vi "Control Example.vi"() -> ()   [LabVIEW 2016]
doc: "Demonstrates the Control Menu type. Right click on the \"Listbox\" to see the menu generated.\n\nClick summarys show up in the history array. Click the \"Add Item\" to add a dummy item to the control's menu."
uses:
  <userlib>/_MGI/Menu Building/SelectionType/RadioSelection/MGI_RadioSelection.lvclass
  C:/Program Files (x86)/National Instruments/LabVIEW 2016/user.lib/_MGI/Menu Building/SelectionType/MGI_SelectionType.lvclass
  <userlib>/_MGI/Menu Building/SelectionType/CheckmarkSelection/MGI_CheckmarkSelection.lvclass
  <userlib>/_MGI/Menu Building/MenuItem/MenuSeparatorItem/MGI_MenuSeparatorItem.lvclass
  C:/Program Files (x86)/National Instruments/LabVIEW 2016/user.lib/_MGI/Menu Building/MenuItem/MGI_MenuItem.lvclass
  <userlib>/_MGI/Menu Building/MenuTypes/Control/MGI_Control.lvclass
  C:/Program Files (x86)/National Instruments/LabVIEW 2016/user.lib/_MGI/Menu Building/MenuTypes/MGI_Menu.lvclass
  <userlib>/_MGI/Menu Building/MenuItem/MenuItem.vi
  <userlib>/_MGI/Menu Building/SelectionType/RadioSelection/RadioSelection.vi
  <userlib>/_MGI/Menu Building/MenuItem/Write Click By Default.vi
  <userlib>/_MGI/Menu Building/MenuItem/Write Sub-Menus.vi
  <userlib>/_MGI/Menu Building/MenuTypes/Control/Control.vi
  <userlib>/_MGI/Menu Building/SelectionType/CheckmarkSelection/CheckmarkSelection.vi
  <userlib>/_MGI/Menu Building/MenuItem/MenuSeparatorItem/MenuSeparatorItem.vi
  <userlib>/_MGI/Menu Building/MenuTypes/Read Menu Items.vi
  <userlib>/_MGI/Menu Building/MenuItem/MGI_MenuItem.lvclass
  <userlib>/_MGI/Menu Building/SelectionType/MGI_SelectionType.lvclass
  <userlib>/_MGI/Menu Building/MenuTypes/MGI_Menu.lvclass
  <userlib>/_MGI/Menu Building/MenuItemStatusChange/MGI_MenuItemStatusChange.lvclass
panel:
  out "History 2":T1(array[cluster])
  in  "Listbox 2":i32(listbox)
  out "History":T1(array[cluster])
  in  "Add Item":bool
  in  "stop":bool
  in  "Listbox":i32(listbox)
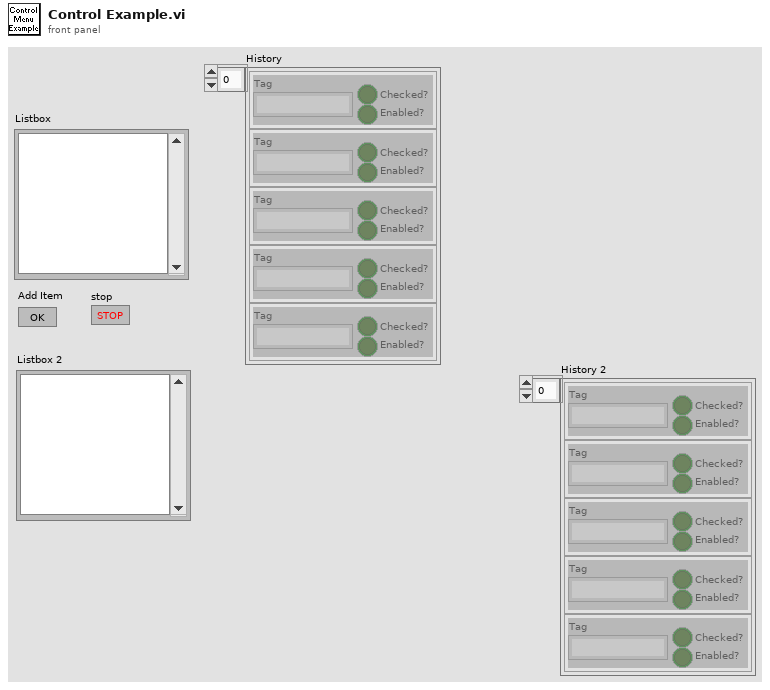
[diagram p1: front panel]
types:
  T1 = cluster{"Tag":string, "Checked?":bool, "Enabled?":bool}[]
  T2 = cluster{"Tag":string, "Checked?":bool, "Enabled?":bool}
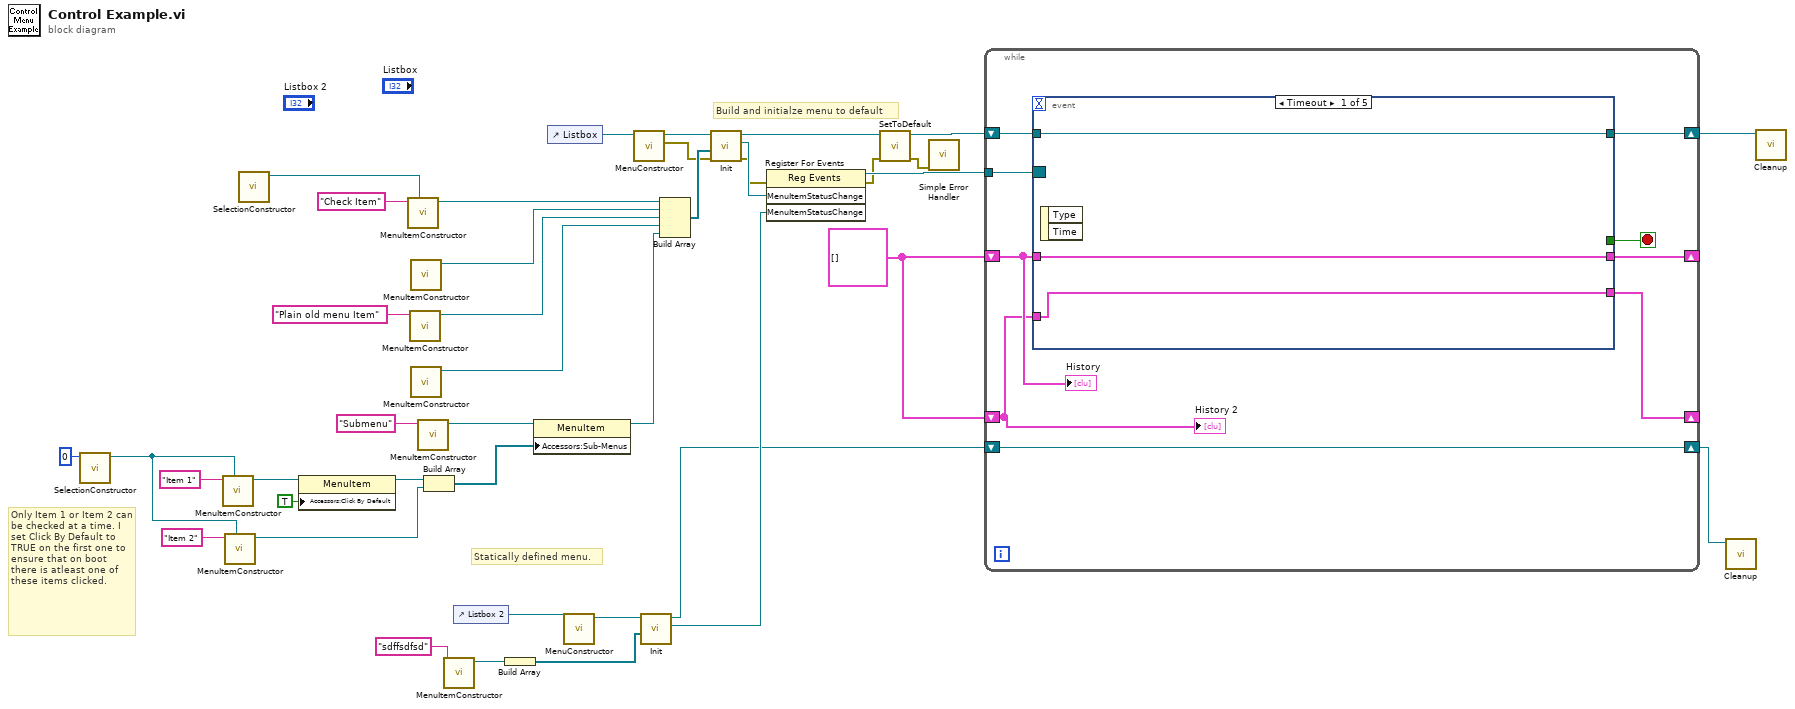
[diagram p0: block diagram]
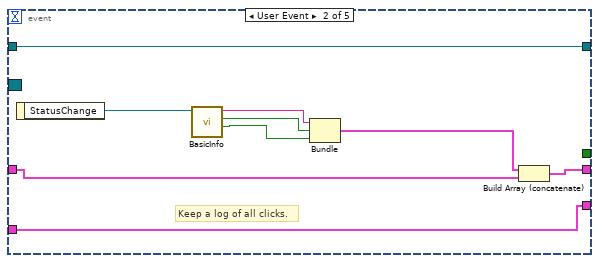
[diagram p2: hidden frame]
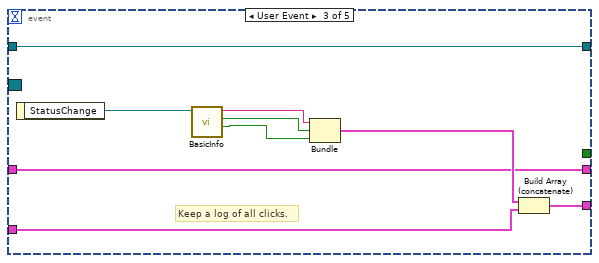
[diagram p3: hidden frame]
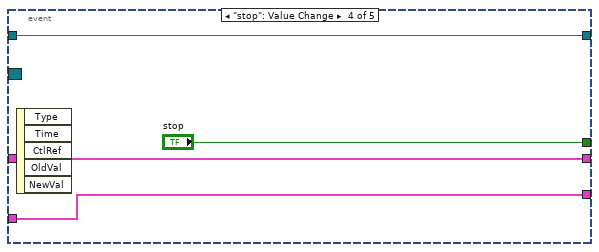
[diagram p4: hidden frame]
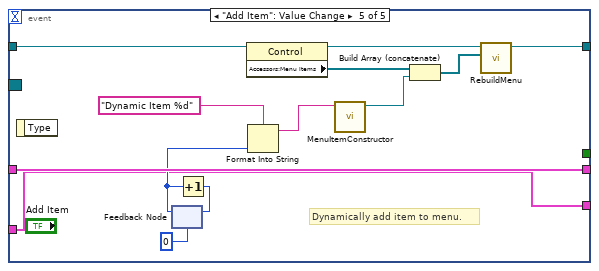
[diagram p5: hidden frame]
diagram:
  w7 = T1 [] ("Array")
  # "Build and initialze menu to default"
  # "Only Item 1 or Item 2 can be checked at a time. I set Click By Default to TRUE on the first one to ensure that on boot there is atleast one of these items clicked."
  # "Statically defined menu."
  n1 = call-poly <userlib>:"SelectionConstructor.vi"("Group"=u8 0) -> ("RadioSelection out"=w26:refnum<class "MGI_RadioSelection.lvclass">)  [unwired: 9 in, 1 out]
  n2 = call-poly <userlib>:"MenuItemConstructor.vi"("Selection Type"=w26, "Text"="Item 1") -> ("MenuItem"=w29:refnum<data-value>)  [unwired: 8 in, 1 out]
  n3 = call-poly <userlib>:"MenuItemConstructor.vi"("Selection Type"=w26, "Text"="Item 2") -> ("MenuItem"=w28:refnum<data-value>)  [unwired: 8 in, 1 out]
  n4 = call-poly <userlib>:"SelectionConstructor.vi"() -> ("CheckmarkSelection out"=w35:refnum<class "MGI_CheckmarkSelection.lvclass">)  [unwired: 10 in, 1 out]
  n5 = property class="MenuItem"(reference=w29, "Accessors:Click By Default"=TRUE ("Click By Default")) -> (reference out=w21:refnum<data-value>)  [unwired: 1 in, 1 out]
  n6 = call-poly <userlib>:"MenuItemConstructor.vi"("Selection Type"=w35, "Text"="Check Item") -> ("MenuItem"=w37:refnum<data-value>)  [unwired: 8 in, 1 out]
  n7 = call-poly <userlib>:"MenuItemConstructor.vi"("Text"="Plain old menu Item") -> ("MenuItem"=w1:refnum<data-value>)  [unwired: 9 in, 1 out]
  n8 = call-poly <userlib>:"MenuItemConstructor.vi"() -> ("MenuSeparatorItem"=w22:refnum<data-value>)  [unwired: 10 in, 1 out]
  n9 = call-poly <userlib>:"MenuItemConstructor.vi"() -> ("MenuSeparatorItem"=w3:refnum<data-value>)  [unwired: 10 in, 1 out]
  n10 = call-poly <userlib>:"MenuItemConstructor.vi"("Text"="Submenu") -> ("MenuItem"=w32:refnum<data-value>)  [unwired: 9 in, 1 out]
  n11 = Build Array(w21, w28) -> (w27:refnum<data-value>[])
  n12 = call-poly <userlib>:"MenuItemConstructor.vi"("Text"="sdffsdfsd") -> ("MenuItem"=w10:refnum<data-value>)  [unwired: 9 in, 1 out]
  n13 = control-ref of="Listbox 2"() -> (w14:refnum<vi>)
  n14 = Build Array(w10) -> (w9:refnum<data-value>[])
  n15 = property class="MenuItem"(reference=w32, "Accessors:Sub-Menus"=w27) -> (reference out=w33:refnum<data-value>)  [unwired: 1 in, 1 out]
  n16 = control-ref of="Listbox"() -> (w24:refnum<vi>)
  n17 = call-poly <userlib>:"MenuConstructor.vi"("Ctl Refnum"=w14) -> ("Control out"=w15:refnum<class "MGI_Control.lvclass">)  [unwired: 9 in, 1 out]
  n18 = call-poly <userlib>:"MenuConstructor.vi"("Ctl Refnum"=w24) -> ("error out"=w6:errorcluster, "Control out"=w23:refnum<class "MGI_Control.lvclass">)  [unwired: 9 in]
  n19 = call-dynamic "Init.vi"("Menu Items"=w9, "Menu in"=w15) -> ("MenuItemStatusChange"=w13:refnum<user-event>, "Menu out"=w12:refnum<class "MGI_Control.lvclass">)  [unwired: 7 in, 1 out]
  n20 = Build Array(w37, w22, w1, w3, w33) -> (w40:refnum<data-value>[])
  n21 = call-dynamic "Init.vi"("error in (no error)"=w6, "Menu Items"=w40, "Menu in"=w23) -> ("error out"=w5:errorcluster, "MenuItemStatusChange"=w39:refnum<user-event>, "Menu out"=w19:refnum<class "MGI_Control.lvclass">)  [unwired: 6 in]
  n22 = register-events(error in=w5, w39, w13) -> (reference out=w38:refnum<event-registration>, error out=w17:errorcluster)  [unwired: 1 in]
  n23 = call-dynamic "SetToDefault.vi"("error in (no error)"=w17, "Menu in"=w19) -> ("error out"=w4:errorcluster, "Menu out"=w18:refnum<class "MGI_Control.lvclass">)  [unwired: 8 in]
  n24 = call <vilib>:"Simple Error Handler.vi"("error in (no error)"=w4) -> ()  [unwired: 4 in, 5 out]
  n25 = while {
    tunnel: w38 -> [w47]
    shift-right: [w46] -> _
    shift-left: w7 -> [w44]
    shift-right: [w45] -> w16
    shift-left: w18 -> [w48]
    shift-right: [w43] -> w11
    shift-left: w12 -> [w43]
    shift-right: [w41] -> _
    shift-left: w7 -> [w42]
    stop <- w49 stop-if-true
    n26 = event shown="[0] Timeout" {
      selector: w47 -> [_ _ _ _ _]
      dyn-events: _ -> [_ _ _ _ _]
      timeout: _ -> [_ _ _ _ _]
      tunnel: [_ _ _ "stop" _] -> w49
      tunnel: w48 -> [w51 w59 w70 w72 w86]
      tunnel: [w52 w61 w62 w73 w87] -> w46
      tunnel: w44 -> [w52 w60 w62 w73 w87]
      tunnel: [w51 w59 w70 w72 w85] -> w45
      tunnel: w42 -> [w50 w53 w64 w71 w75]
      tunnel: [w50 w53 w63 w71 w75] -> w41
      event Timeout {
        n27 = event-data() -> ()  [unwired: 1 in, 2 out]
      }
      event User Event {
        # "Keep a log of all clicks."
        n28 = event-data() -> ("StatusChange"=w58:refnum<class "MGI_MenuItemStatusChange.lvclass">)  [unwired: 1 in]
        n29 = call <userlib>:"BasicInfo.vi"("MGI_MenuItemStatusChange in"=w58) -> ("Enabled?"=w55:bool, "Checked?"=w56:bool, "Tag"=w57:string)  [unwired: 7 in, 1 out]
        n30 = Bundle("Tag"=w57, "Checked?"=w56, "Enabled?"=w55) -> (w54:T2)  [unwired: 1 in]
        n31 = Build Array (concatenate)(w54, w60) -> (w61:T1)
      }
      event User Event {
        # "Keep a log of all clicks."
        n32 = event-data() -> ("StatusChange"=w69:refnum<class "MGI_MenuItemStatusChange.lvclass">)  [unwired: 1 in]
        n33 = call <userlib>:"BasicInfo.vi"("MGI_MenuItemStatusChange in"=w69) -> ("Enabled?"=w66:bool, "Checked?"=w67:bool, "Tag"=w68:string)  [unwired: 7 in, 1 out]
        n34 = Bundle("Tag"=w68, "Checked?"=w67, "Enabled?"=w66) -> (w65:T2)  [unwired: 1 in]
        n35 = Build Array (concatenate)(w65, w64) -> (w63:T1)
      }
      event "stop": Value Change {
        n36 = event-data() -> ()  [unwired: 1 in, 5 out]
      }
      event "Add Item": Value Change {
        # "Dynamically add item to menu."
        n37 = event-data() -> ()  [unwired: 1 in, 1 out]
        n38 = feedback #1(0) -> (w78:i32)
        n39 = Increment(x=w78) -> (x+1=w77:i32)
        n40 = feedback-in #1(w77) -> ()
        n41 = property class="Control"(reference=w86) -> (reference out=w84:refnum<class "MGI_Control.lvclass">, "Accessors:Menu Items"=w83:refnum<data-value>[])  [unwired: 1 in, 1 out]
        n42 = Format Into String(format string="Dynamic Item %d" ("Text"), w78) -> (resulting string=w76:string)  [unwired: 2 in, 1 out]
        n43 = call-poly <userlib>:"MenuItemConstructor.vi"("Text"=w76) -> ("MenuItem"=w81:refnum<data-value>)  [unwired: 9 in, 1 out]
        n44 = Build Array (concatenate)(w83, w81) -> (w82:refnum<data-value>[])
        n45 = call <userlib>:"RebuildMenu.vi"("New Menu Items"=w82, "Menu in"=w84) -> ("Menu out"=w85:refnum<class "MGI_Control.lvclass">)  [unwired: 8 in, 1 out]
      }
    }
    "History" <- w44
    "History 2" <- w42
  }
  n46 = call-dynamic "Cleanup.vi"("Control in"=w11) -> ()  [unwired: 10 in, 1 out]
  n47 = call-dynamic "Cleanup.vi"("Control in"=w16) -> ()  [unwired: 10 in, 1 out]
